vi "纳清电导率_所有参数读取.vi"(8 "error in (no error)":errorcluster caption="错误输入（无错误）", 11 "MB session in":refnum<class "MB_Master.lvclass">) -> (0 "error out":errorcluster caption="错误输出", 2 "输出值":T1 {"波特率" items=["4800", "9600", "19200", "38400", "57600", "115200"]}, 3 "MB session out":refnum<class "MB_Master.lvclass">)   [LabVIEW 2016, in "斯坦道多参数.lvlib"]
uses:
  <vilib>/Plasmionique/MB Master/MB_Master/MB_Master.lvclass
  <vilib>/Plasmionique/MB Master/MB Master.lvlib
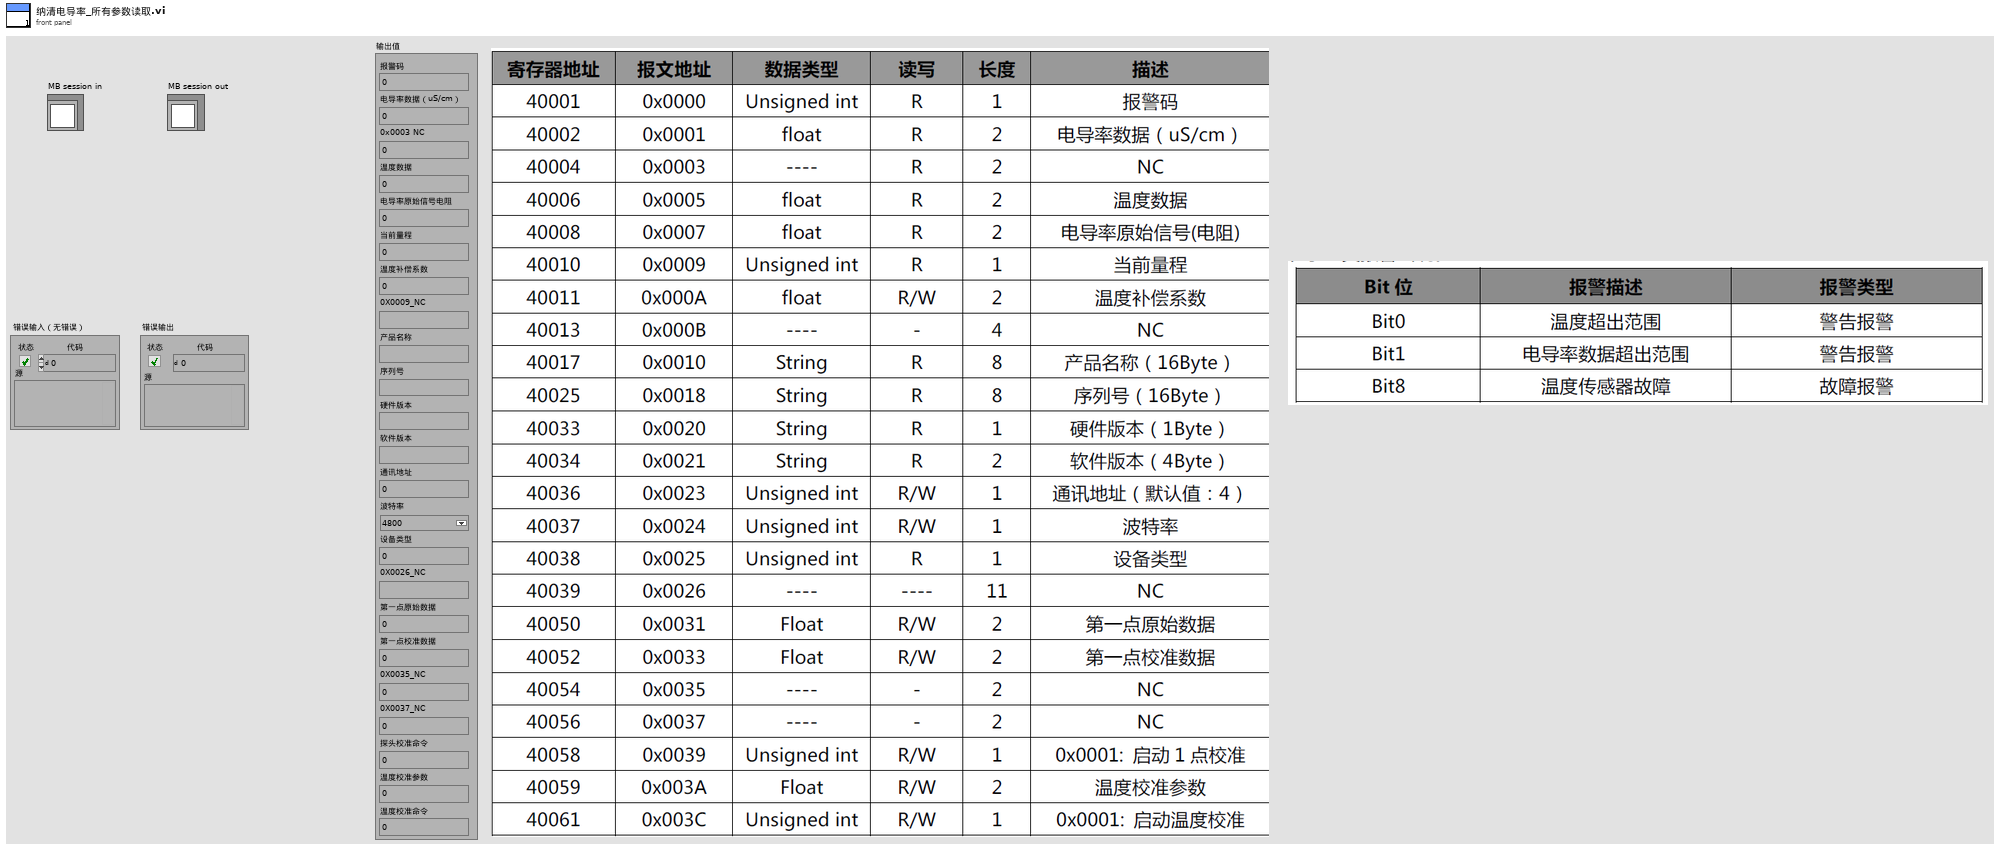
[diagram p1: front panel]
types:
  T1 = cluster{"报警码":u16, "电导率数据（uS/cm）":sgl, "0x0003 NC":sgl, "温度数据":sgl, "电导率原始信号电阻":sgl, "当前量程":u16, "温度补偿系数":sgl, "0X0009_NC":string, "产品名称":string, "序列号":string, "硬件版本":string, "软件版本":string, "通讯地址":u16, "波特率":u16, "设备类型":u16, "0X0026_NC":string, "第一点原始数据":sgl, "第一点校准数据":sgl, "0X0035_NC":sgl, "0X0037_NC":sgl, "探头校准命令":u16, "温度校准参数":sgl, "温度校准命令":u16}
  T2 = cluster{u16, "数值":sgl, "数值":sgl, "数值":sgl, "数值":sgl, u16, "数值":sgl, "类型":string, "类型":string, "类型":string, "类型":string, "类型":string, u16, u16, u16, "类型":string, "数值":sgl, "数值":sgl, "数值":sgl, "数值":sgl, u16, "数值":sgl, u16}
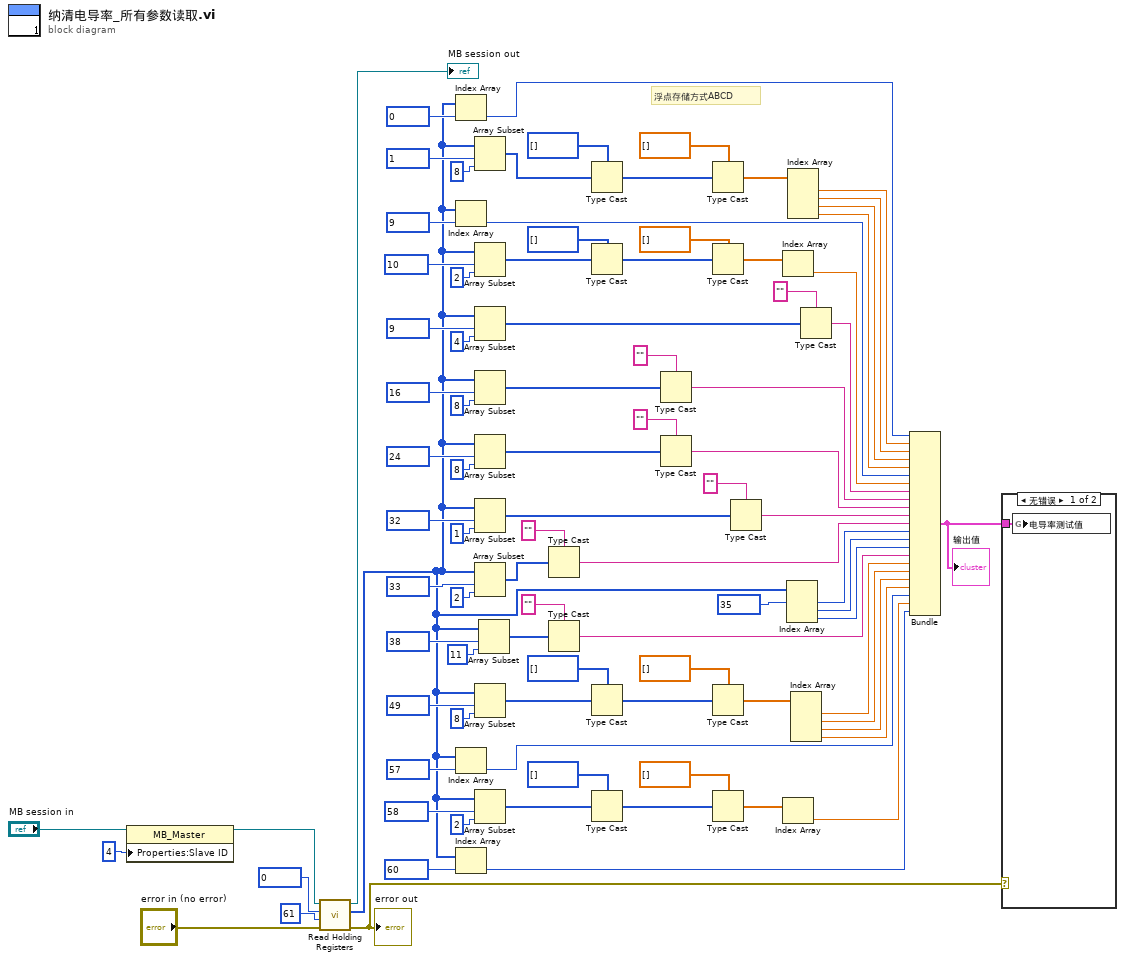
[diagram p0: block diagram]
diagram:
  # "浮点存储方式ABCD"
  n1 = property class="MB_Master"(reference="MB session in", "Properties:Slave ID"=u8 4 ("Slave ID")) -> (reference out=w80:refnum<class "MB_Master.lvclass">)  [unwired: 1 in, 1 out]
  n2 = call <vilib>:"Read Holding Registers.vi"("error in (no error)"="error in (no error)", "quantity"=u16 61, "starting address"=u16 0, "MB session in"=w80) -> ("error out"=w21:errorcluster, "Registers"=w2:u16[], "MB session out"=→"MB session out":refnum<class "MB_Master.lvclass">)  [unwired: 5 in]
  "error out" <- w21
  n3 = Index Array(array=w2, index=u16 0 ("starting address")) -> (element=w88:u16)
  n4 = Index Array(array=w2, index=u16 9 ("starting address")) -> (element=w1:u16)
  n5 = Index Array(array=w2, index=u16 57 ("starting address")) -> (element=w25:u16)
  n6 = Index Array(array=w2, index=u16 60 ("starting address")) -> (element=w22:u16)
  n7 = Array Subset(array=w2, index=u16 1 ("starting address"), length=8 ("长度")) -> (w84:u16[])
  n8 = Array Subset(array=w2, index=u16 10 ("starting address"), length=2 ("长度")) -> (w5:u16[])
  n9 = Array Subset(array=w2, index=u16 9 ("starting address"), length=4 ("长度")) -> (w73:u16[])
  n10 = Array Subset(array=w2, index=u16 16 ("starting address"), length=8 ("长度")) -> (w69:u16[])
  n11 = Array Subset(array=w2, index=u16 24 ("starting address"), length=8 ("长度")) -> (w63:u16[])
  n12 = Array Subset(array=w2, index=u16 32 ("starting address"), length=1 ("长度")) -> (w59:u16[])
  n13 = Array Subset(array=w2, index=u16 33 ("starting address"), length=2 ("长度")) -> (w53:u16[])
  n14 = Array Subset(array=w2, index=u16 49 ("starting address"), length=8 ("长度")) -> (w40:u16[])
  n15 = Array Subset(array=w2, index=u16 58 ("starting address"), length=2 ("长度")) -> (w28:u16[])
  n16 = Array Subset(array=w2, index=u16 38 ("starting address"), length=11 ("长度")) -> (w43:u16[])
  n17 = Type Cast(type="" ("类型"), x=w53) -> (*(type *) &x=w51:string)
  n18 = Type Cast(type="" ("类型"), x=w43) -> (*(type *) &x=w42:string)
  n19 = Type Cast(type=u32[] [] ("数组 2"), x=w84) -> (*(type *) &x=w20:u32[])
  n20 = Type Cast(type=u32[] [] ("数组 2"), x=w5) -> (*(type *) &x=w9:u32[])
  n21 = Type Cast(type=u32[] [] ("数组 2"), x=w40) -> (*(type *) &x=w38:u32[])
  n22 = Type Cast(type=u32[] [] ("数组 2"), x=w28) -> (*(type *) &x=w30:u32[])
  n23 = Type Cast(type="" ("类型"), x=w69) -> (*(type *) &x=w66:string)
  n24 = Type Cast(type="" ("类型"), x=w63) -> (*(type *) &x=w61:string)
  n25 = Type Cast(type=sgl[] [] ("数组 2"), x=w20) -> (*(type *) &x=w83:sgl[])
  n26 = Type Cast(type=sgl[] [] ("数组 2"), x=w9) -> (*(type *) &x=w8:sgl[])
  n27 = Type Cast(type=sgl[] [] ("数组 2"), x=w38) -> (*(type *) &x=w35:sgl[])
  n28 = Type Cast(type=sgl[] [] ("数组 2"), x=w30) -> (*(type *) &x=w33:sgl[])
  n29 = Type Cast(type="" ("类型"), x=w59) -> (*(type *) &x=w56:string)
  n30 = Index Array(array=w8) -> (element=w4:sgl)  [unwired: 1 in]
  n31 = Index Array(array=w33) -> (element=w24:sgl)  [unwired: 1 in]
  n32 = Index Array(array=w2, index #1=u16 35 ("starting address")) -> (element #1=w49:u16, element #2=w48:u16, element #3=w47:u16)  [unwired: 2 in]
  n33 = Index Array(array=w83) -> (element #1=w78:sgl, element #2=w77:sgl, element #3=w17:sgl, element #4=w16:sgl)  [unwired: 4 in]
  n34 = Index Array(array=w35) -> (element #1=w34:sgl, element #2=w15:sgl, element #3=w14:sgl, element #4=w13:sgl)  [unwired: 4 in]
  n35 = Type Cast(type="" ("类型"), x=w73) -> (*(type *) &x=w71:string)
  n36 = Bundle(w88, "数值"=w78, "数值"=w77, "数值"=w17, "数值"=w16, w1, "数值"=w4, "类型"=w71, "类型"=w66, "类型"=w61, "类型"=w56, "类型"=w51, w49, w48, w47, "类型"=w42, "数值"=w34, "数值"=w15, "数值"=w14, "数值"=w13, w25, "数值"=w24, w22) -> (w12:T2)  [unwired: 1 in]
  "输出值" <- w12
  n37 = case shown="无错误" w21 {
    tunnel: w12 -> [w91 _]
    frame No Error {
      n38 = global write "纳清过程全局变量.vi" "电导率测试值"(w91) -> ()
    }
    frame Error {
    }
  }
